vi "Project_Labview.vi"() -> ()   [LabVIEW 2025]
uses:
  <vilib>/Instr/_visa.llb/VISA Configure Serial Port (Instr).vi
  <vilib>/ptbypt/NI_PtbyPt.lvlib
panel:
  out "Angle History":dbl(graph)
  out "Distance":dbl
  out "Right Motor PWM":dbl(knob) scale=-255.0..255.0
  out "Left Motor PWM":dbl(knob) scale=-255.0..255.0
  out "Tilt Angle":dbl(knob) scale=-45.0..45.0
  in  "Stop Simulation":bool
  in  "Arduino Port":refnum<visa-resource-name>
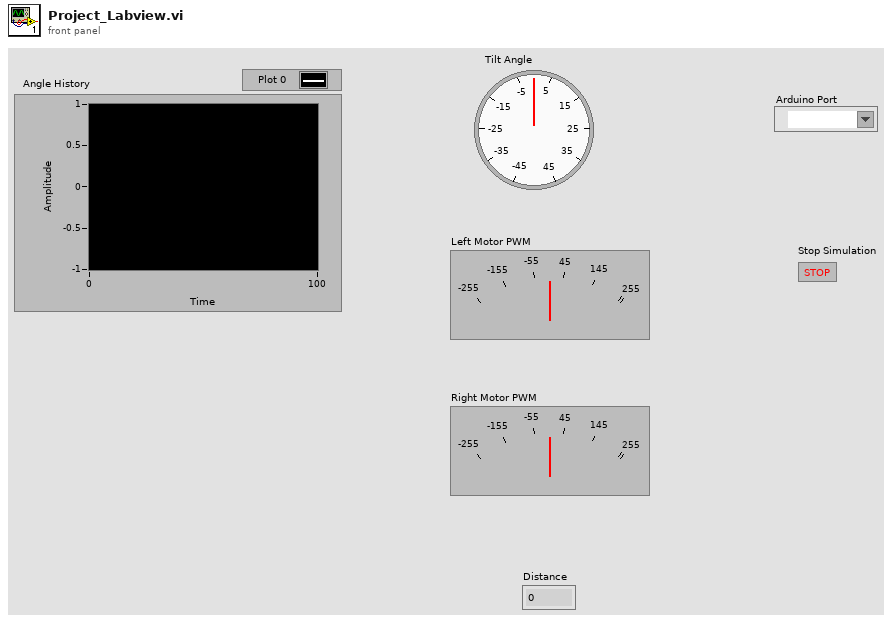
[diagram p1: front panel]
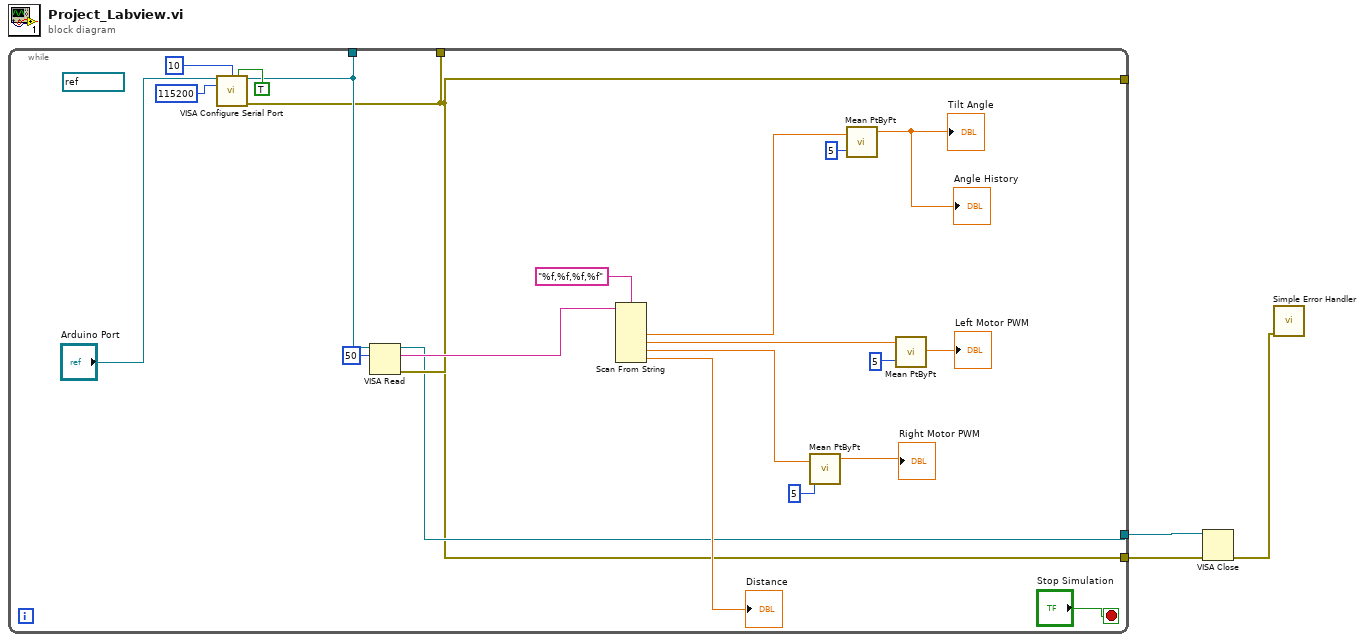
[diagram p0: block diagram]
diagram:
  n1 = while {
    tunnel: [w8] -> _
    tunnel: [w7] -> _
    tunnel: [w7] -> _
    tunnel: [w6] -> w3
    tunnel: [w5] -> w2
    stop <- "Stop Simulation" stop-if-true
    (unwired) refnum<visa-resource-name> "COM3" ("VISA resource name")
    n2 = call-poly "VISA Configure Serial Port"("VISA resource name"="Arduino Port", "termination char\n(0xA = '\\n' = LF)"=u8 10 ("termination char\n(0xA = '\\n' = LF)"), "Enable Termination\nChar (T)"=TRUE ("Enable Termination\nChar (T)"), "baud rate (9600)"=u32 115200) -> ("VISA resource name out"=w8:refnum<visa-resource-name>, "error out"=w7:errorcluster)  [unwired: 10 in]
    n3 = VISA Read(VISA resource name=w8, byte count=u32 50, error in (no error)=w7) -> (VISA resource name out=w6:refnum<visa-resource-name>, read buffer=w20:string, error out=w5:errorcluster)  [unwired: 1 out]
    n4 = Scan From String(format string="%f,%f,%f,%f", input string=w20) -> (output 1=w15:dbl, output 2=w13:dbl, output 3=w11:dbl, output 4=→"Distance":dbl)  [unwired: 6 in, 3 out]
    n5 = call <vilib>:"Mean PtByPt.vi"("x"=w11, "sample length"=5) -> ("mean"=→"Right Motor PWM":dbl)  [unwired: 2 in, 1 out]
    n6 = call <vilib>:"Mean PtByPt.vi"("x"=w15, "sample length"=5) -> ("mean"=→"Tilt Angle" →"Angle History":dbl)  [unwired: 2 in, 1 out]
    n7 = call <vilib>:"Mean PtByPt.vi"("x"=w13, "sample length"=5) -> ("mean"=→"Left Motor PWM":dbl)  [unwired: 2 in, 1 out]
  }
  n8 = VISA Close(VISA resource name=w3, error in (no error)=w2) -> (error out=w1:errorcluster)
  n9 = call <vilib>:"Simple Error Handler.vi"("error in (no error)"=w1) -> ()  [unwired: 4 in, 5 out]
